vi "CalculoTesteQuadrada_Validacao.vi"(8 "Tempo":dbl, 9 "RPM":dbl, 10 "Min":dbl, 11 "Max":dbl) -> (3 "XY Graph":cluster{"X":dbl, "Y":dbl}[](graph))   [LabVIEW 2019]
uses:
  <vilib>/Analysis/NI_AAL_SigProc.lvlib
panel:
  in  "Tempo b subida":dbl
  in  "Tempo b descida":dbl
  out "Array":dbl[](array[numeric])
  # "Max: 60 pontos por segundo"
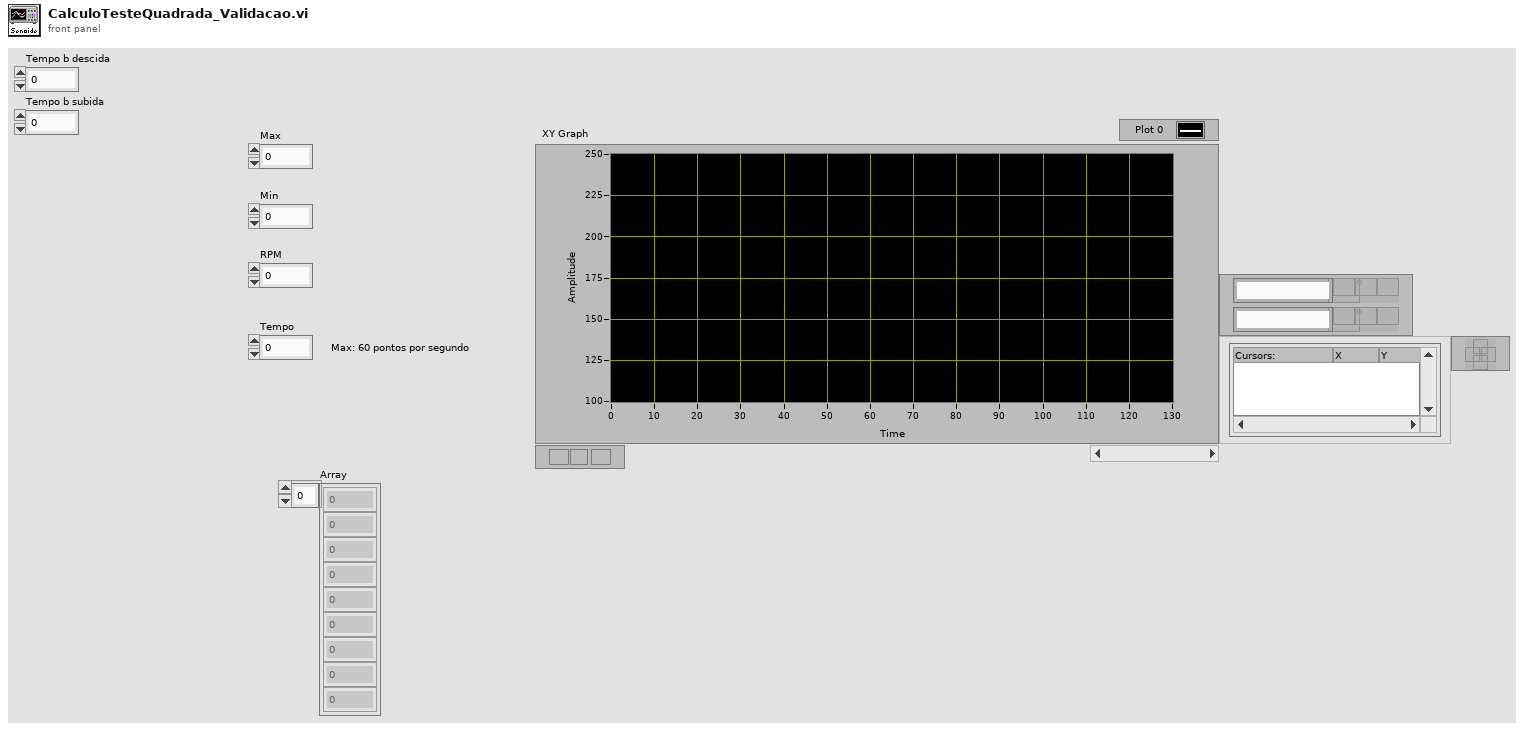
[diagram p1: front panel]
types:
  T1 = cluster{"Frequencia":dbl, "Fase":dbl, "AmplitudeOnda":dbl, "Offset":dbl, "Tempo b subida":dbl, "Tempo b descida":dbl}
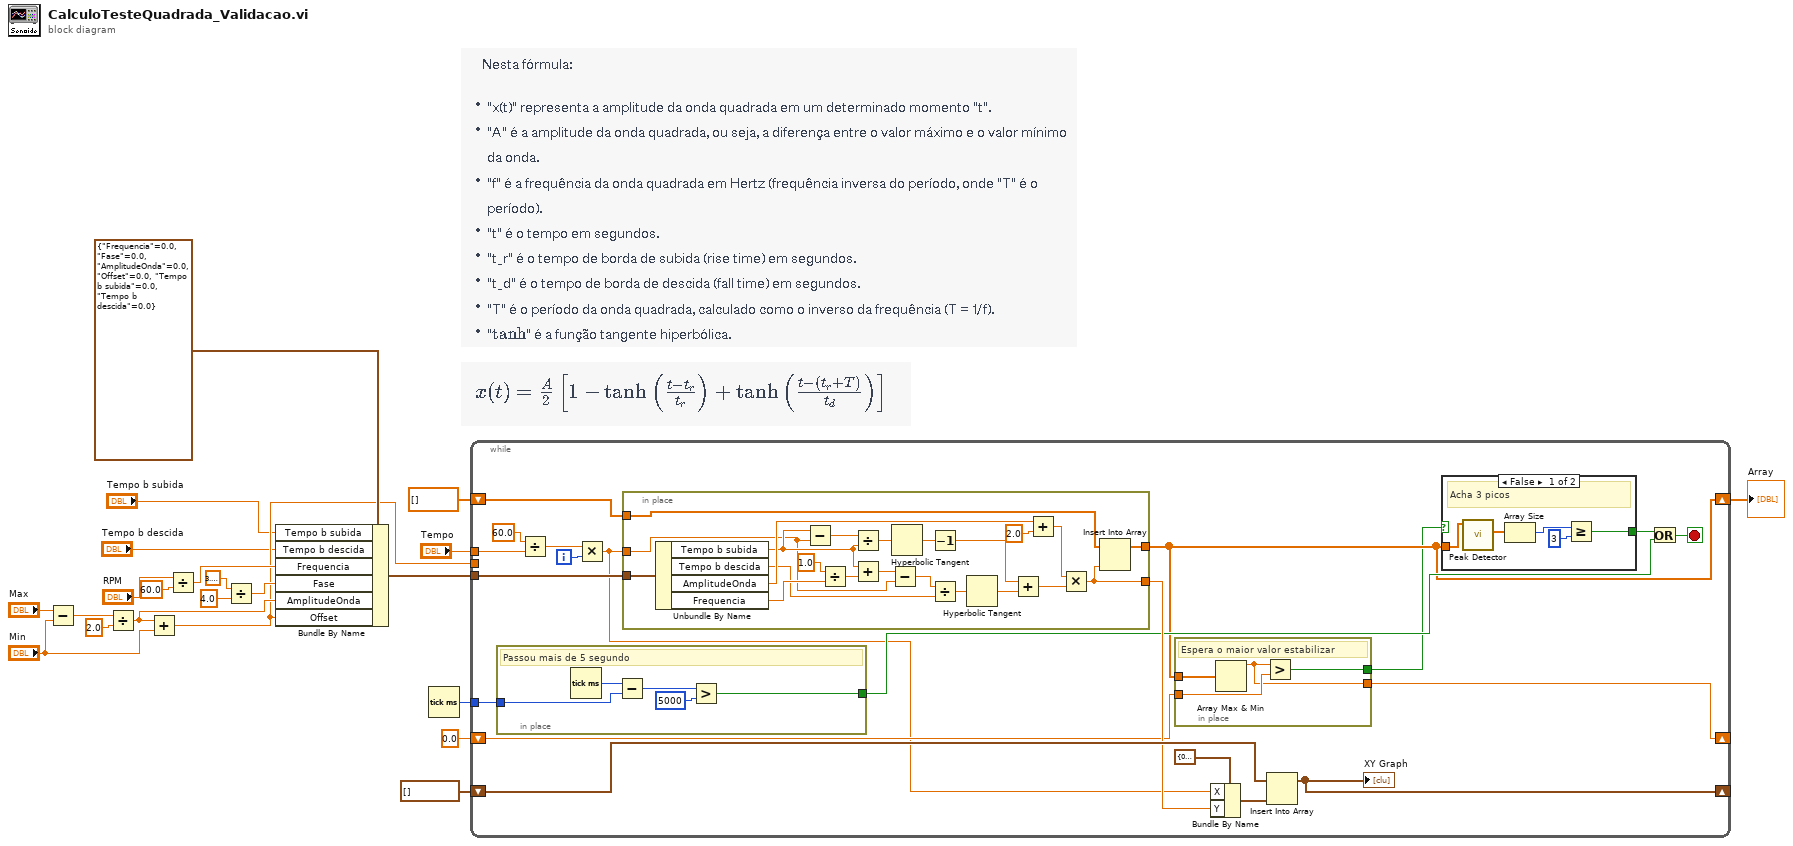
[diagram p0: block diagram]
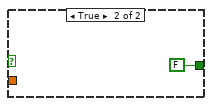
[diagram p2: hidden frame]
diagram:
  n1 = Subtract(x="Max", y="Min") -> (x-y=w13:dbl)
  n2 = Divide(x=w13, y=2.0) -> (x/y=w8:dbl)
  n3 = Add(x=w8, y="Min") -> (x+y=w3:dbl)
  n4 = Divide(x="RPM", y=60.0) -> (x/y=w10:dbl)
  n5 = Divide(x=3.141592653589793, y=4.0) -> (x/y=w9:dbl)
  n6 = Bundle By Name(cluster=T1 {"Frequencia"=0.0, "Fase"=0.0, "AmplitudeOnda"=0.0, "Offset"=0.0, "Tempo b subida"=0.0, "Tempo b descida"=0.0}, "Tempo b subida"="Tempo b subida", "Tempo b descida"="Tempo b descida", "Frequencia"=w10, "Fase"=w9, "AmplitudeOnda"=w8, "Offset"=w3) -> (w7:T1)
  n7 = Tick Count (ms)() -> (millisecond timer value=w14:u32)
  n8 = while {
    shift-right: [w33] -> w4
    shift-left: dbl[] [] -> [w34]
    shift-right: [w41] -> _
    shift-left: cluster{"X":dbl, "Y":dbl}[] [] ("GraphSenoide") -> [w42]
    tunnel: w14 -> [w37]
    shift-right: [w30] -> _
    shift-left: 0.0 -> [w32]
    tunnel: w7 -> [w28]
    tunnel: "Tempo" -> [w26]
    tunnel: w3 -> [_]
    i -> [w24]
    stop <- w35 stop-if-true
    n9 = in-place {
      in-place-border: w37 -> [w79]
      in-place-border: [w75] -> w36
      # "Passou mais de 5 segundo"
      n10 = Tick Count (ms)() -> (millisecond timer value=w78:u32)
      n11 = Subtract(x=w78, y=w79) -> (x-y=w77:u32)
      n12 = Greater?(x=w77, y=u32 5000) -> (0:w75:bool)
    }
    n13 = Divide(x=60.0, y=w26) -> (x/y=w25:dbl)
    n14 = Multiply(x=w25, y=w24) -> (x*y=w23:dbl)
    n15 = in-place {
      in-place-border: [w58] -> w38
      in-place-border: w34 -> [w64]
      in-place-border: [w63] -> w33
      in-place-border: w28 -> [w62]
      in-place-border: w23 -> [w49]
      n16 = Unbundle By Name(w62) -> ("Tempo b subida"=w53:dbl, "Tempo b descida"=w46:dbl, "AmplitudeOnda"=w61:dbl, "Frequencia"=w51:dbl)
      n17 = Subtract(x=w53, y=w49) -> (x-y=w57:dbl)
      n18 = Divide(x=1.0, y=w51) -> (x/y=w50:dbl)
      n19 = Divide(x=w57, y=w53) -> (x/y=w56:dbl)
      n20 = Add(x=w53, y=w50) -> (x+y=w48:dbl)
      n21 = Subtract(x=w48, y=w49) -> (x-y=w47:dbl)
      n22 = Hyperbolic Tangent(1:w56) -> (0:w55:dbl)
      n23 = Decrement(x=w55) -> (x-1=w54:dbl)
      n24 = Divide(x=w47, y=w46) -> (x/y=w45:dbl)
      n25 = Hyperbolic Tangent(1:w45) -> (0:w44:dbl)
      n26 = Add(x=w54, y=w44) -> (x+y=w43:dbl)
      n27 = Add(x=w61, y=2.0) -> (x+y=w59:dbl)
      n28 = Multiply(x=w59, y=w43) -> (x*y=w58:dbl)
      n29 = Insert Into Array(array=w64, new element=w58) -> (w63:dbl[])  [unwired: 1 in]
    }
    n30 = in-place {
      in-place-border: w33 -> [w68]
      in-place-border: w32 -> [w67]
      in-place-border: [w66] -> w31
      in-place-border: [w65] -> w30
      # "Espera o maior valor estabilizar"
      n31 = Array Max & Min(array=w68) -> (max value=w65:dbl)  [unwired: 3 out]
      n32 = Greater?(x=w65, y=w67) -> (0:w66:bool)
    }
    n33 = Bundle By Name(cluster=cluster{"X":dbl, "Y":dbl} {"X"=0.0, "Y"=0.0} ("new element/subarray"), "X"=w23, "Y"=w38) -> (w39:cluster{"X":dbl, "Y":dbl})
    n34 = Insert Into Array(array=w42, new element=w39) -> (w41:cluster{"X":dbl, "Y":dbl}[])  [unwired: 1 in]
    "XY Graph" <- w41
    n35 = case shown="False" w31 {
      tunnel: w33 -> [w73 _]
      tunnel: [w69 FALSE] -> w29
      frame False {
        # "Acha 3 picos"
        n36 = call <vilib>:"Peak Detector.vi"("X"=w73) -> ("Amplitudes"=w70:dbl[])  [unwired: 6 in, 4 out]
        n37 = Array Size(array=w70) -> (size(s)=w72:i32)
        n38 = Greater Or Equal?(x=w72, y=3) -> (x >= y?=w69:bool)
      }
      frame True {
      }
    }
    n39 = Or(x=w29, y=w36) -> (x .or. y?=w35:bool)
  }
  "Array" <- w4
